vi "GetTagListing.vi"(8 "error in (no error)":errorcluster) -> (0 "error out":errorcluster, 2 "info":string[][](array[string]), 3 "tags":string[](array[string]))   [LabVIEW 2019]
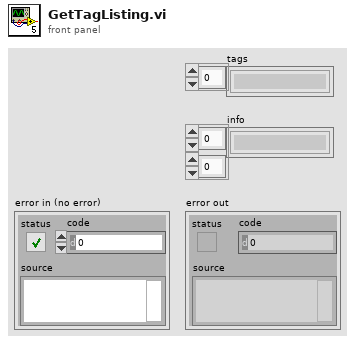
[diagram p1: front panel]
types:
  T1 = enum16{"GET", "PUT", "POST", "MultiPOST", "DELETE"}
  T2 = cluster{"tagsWithValues":cluster{"tag":cluster{"path":string, "type":string}, "current":cluster{"timestamp":string, "value":cluster{"type":string, "value":string}}}[]}
  T3 = cluster{"Name":string, "BaseURL":string, "AppKey":string, "Headers":string[], "Timeout":i32}
  T4 = cluster{"url":string, "sent headers":string, "sent body":string, "headers":string, "body":string, "Sent":string, "Received":string}
  T5 = cluster{"tag":cluster{"path":string, "type":string}, "current":cluster{"timestamp":string, "value":cluster{"type":string, "value":string}}}[]
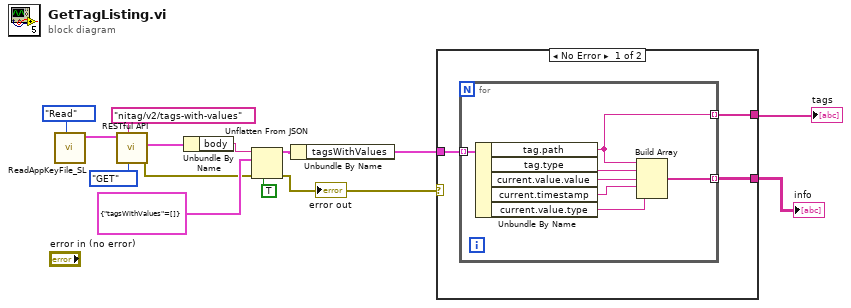
[diagram p0: block diagram]
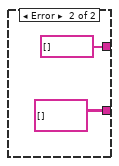
[diagram p2: hidden frame]
diagram:
  n1 = call "ReadAppKeyFile_SL.vi"("Task"=enum16{"Read", "Write"}."Read") -> ("Device Out"=w7:T3)  [unwired: 8 in, 2 out]
  n2 = call "RESTful API.vi"("Method"=T1."GET", "url"="nitag/v2/tags-with-values", "Device In"=w7) -> ("error out"=w10:errorcluster, "Comm"=w9:T4)  [unwired: 6 in, 1 out]
  n3 = Unbundle By Name(w9) -> ("body"=w4:string)
  n4 = Unflatten From JSON(JSON string=w4, type and defaults=T2 {"tagsWithValues"=[]}, default null elements? (F)=TRUE, error in (no error)=w10) -> (value=w1:T2, error out=w5:errorcluster)  [unwired: 3 in]
  "error out" <- w5
  n5 = Unbundle By Name(w1) -> ("tagsWithValues"=w3:T5)
  n6 = case shown="No Error" w5 {
    tunnel: w3 -> [w17 _]
    tunnel: [w16 string[][] []] -> w12
    tunnel: [w15 string[] []] -> w14
    frame No Error {
      n7 = for {
        tunnel: w17 -> [w24] mode=indexing
        tunnel: [w19] -> w16 mode=indexing
        tunnel: [w18] -> w15 mode=indexing
        n8 = Unbundle By Name(w24) -> ("tag.path"=w18:string, "tag.type"=w23:string, "current.value.value"=w22:string, "current.timestamp"=w21:string, "current.value.type"=w20:string)
        n9 = Build Array(w18, w23, w22, w21, w20) -> (w19:string[])
      }
    }
    frame Error {
    }
  }
  "tags" <- w14
  "info" <- w12
